vi "Read RT FIFO.vi"(8 "error in":errorcluster, 11 "RT Data In":refnum<class "DCM-NIVS-RT.lvclass">) -> (0 "error out":errorcluster, 3 "RT Data Out":refnum<class "DCM-NIVS-RT.lvclass">)   [LabVIEW 2016, in "DCM Engine.lvlib"]
uses:
  DCM Engine.lvlib
  Classes/DCM-NIVS-RT/DCM-NIVS-RT.lvclass
  Classes/DCM-NIVS-RT/Device Inputs Write.vi
  Classes/DCM-NIVS-RT/DeviceInFIFO Write.vi
  Classes/DCM-NIVS-RT/Device Inputs Read.vi
  Classes/DCM-NIVS-RT/DeviceInFIFO Read.vi
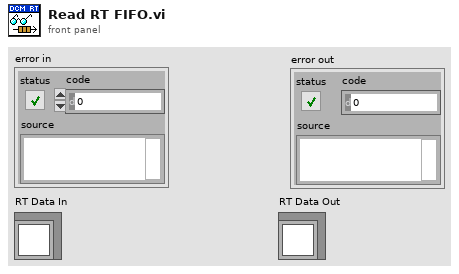
[diagram p1: front panel]
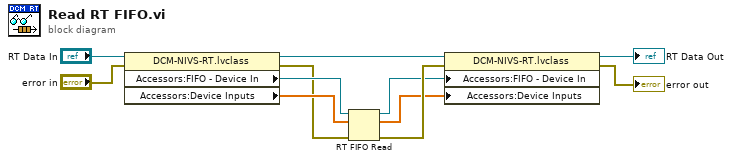
[diagram p0: block diagram]
diagram:
  n1 = property class="DCM-NIVS-RT.lvclass"(reference="RT Data In", error in="error in") -> (reference out=w6:refnum<class "DCM-NIVS-RT.lvclass">, error out=w7:errorcluster, "Accessors:FIFO - Device In"=w9:refnum<k33>, "Accessors:Device Inputs"=w8:dbl[])
  n2 = RT FIFO Read(0:w9, 1:w8, 3:w7) -> (8:w2:refnum<k33>, 9:w1:dbl[], 11:w5:errorcluster)  [unwired: 1 in, 2 out]
  n3 = property class="DCM-NIVS-RT.lvclass"(reference=w6, error in=w5, "Accessors:FIFO - Device In"=w2, "Accessors:Device Inputs"=w1) -> (reference out=→"RT Data Out":refnum<class "DCM-NIVS-RT.lvclass">, error out=→"error out":errorcluster)
